vi "New JSON Object (Multi Numeric).vi"(7 "keys":string[](array[string]), 8 "error in (no error)":errorcluster, 10 "values":dbl[](array[numeric])) -> (0 "error out":errorcluster, 3 "JSON Object out":refnum<class "JSON Object.lvclass">)   [LabVIEW 2016, in "LVJSON.lvlib" / "JSON Object.lvclass"]
doc: "Create a new JSON Object initialized with the given key value pairs. The key and value arrays must be the same size."
uses:
  JSON Object.lvclass
  JSON Numeric/JSON Numeric.lvclass
  C:/Users/tblair/Documents/Git Projects/JSON-Support-for-LabVIEW/Source/JSON Data Classes/JSON Datatype/JSON Null.lvclass
  Insert Key Value Pair (Multi).vi
  JSON Numeric/New JSON Numeric.vi
  JSON Helper/JSON Helper.lvclass
  C:/Users/tblair/Documents/Git Projects/JSON-Support-for-LabVIEW/Source/JSON Data Classes/JSON Basic Type/JSON Literal.lvclass
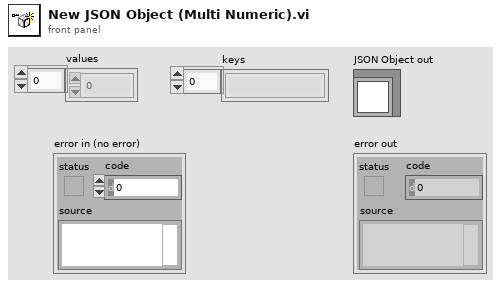
[diagram p1: front panel]
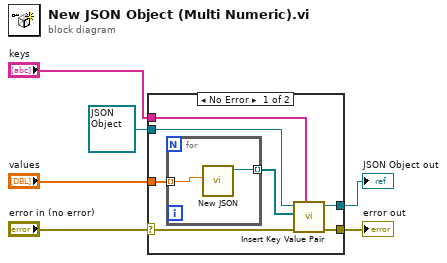
[diagram p0: block diagram]
diagram:
  n1 = case shown="No Error" "error in (no error)" {
    selector: "error in (no error)" -> [w13 w17]
    tunnel: [w12 w17] -> w5
    tunnel: [w10 w16] -> w4
    tunnel: refnum<class "JSON Object.lvclass"> refnum ("JSON Object.lvclass") -> [w11 w16]
    tunnel: "keys" -> [w9 _]
    tunnel: "values" -> [w8 _]
    frame No Error {
      n2 = for {
        tunnel: w8 -> [w15] mode=indexing
        tunnel: [w14] -> w7 mode=indexing
        n3 = call-poly "New JSON.vi"("value"=w15) -> ("JSON String out"=w14:refnum<class "JSON Numeric.lvclass">)  [unwired: 9 in, 1 out]
      }
      n4 = call-poly "Insert Key Value Pair.vi"("keys"=w9, "error in (no error)"=w13, "values"=w7, "JSON Object in"=w11) -> ("error out"=w12:errorcluster, "JSON Object out"=w10:refnum<class "JSON Object.lvclass">)  [unwired: 5 in, 1 out]
    }
    frame Error {
    }
  }
  "error out" <- w5
  "JSON Object out" <- w4
